vi "Get Spectral Map.vi"   [LabVIEW 2017]
doc: "Returns the spectral map of <B>scaled signal [EU]</B>. You can use this polymorphic VI to return <B>spectral map</B> as a 2D array of double-precision, floating-point numbers or a 2D array of 8-bit unsigned integers. You must manually select the polymorphic instance to use. Use the DBL instance to obtain more accurate data. Use the U8 instance to reduce memory usage when the VI displays data."
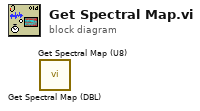
[diagram p0: block diagram]
diagram:
  n1 = call <vilib>:"Get Spectral Map (DBL).vi"() -> ()  [unwired: 7 in, 5 out]
  n2 = call <vilib>:"Get Spectral Map (U8).vi"() -> ()  [unwired: 7 in, 5 out]
